vi "GUILaptop.vi"() -> ()   [LabVIEW 2016]
uses:
  Control/StreamCluster.ctl
  Control/GUICluster.ctl
panel:
  out "Joule":dbl
  out "Rundenzeit":T1
  out "stop 2":bool
  in  "Start":bool
  in  "Stop":bool
  in  "Geschwindigkeit multiplikator":dbl(knob)=0.039196582802747515 scale=0.0..1.0
  out "Linefollow-Array":bool[](array[boolean])
  out "Geschwindigkeit [m/s]":dbl(knob) scale=0.0..4.5
  out "schräg L":dbl format="%#_3g"
  out "schräge R":dbl format="%#_3g"
  out "Strom [A]":dbl(graph)
  out "rechts":dbl format="%#_3g"
  out "links":dbl format="%#_3g"
  out "gerade L":dbl format="%#_3g"
  out "gerade R":dbl format="%#_3g"
  # "Minimum"
  # "Gesamt"
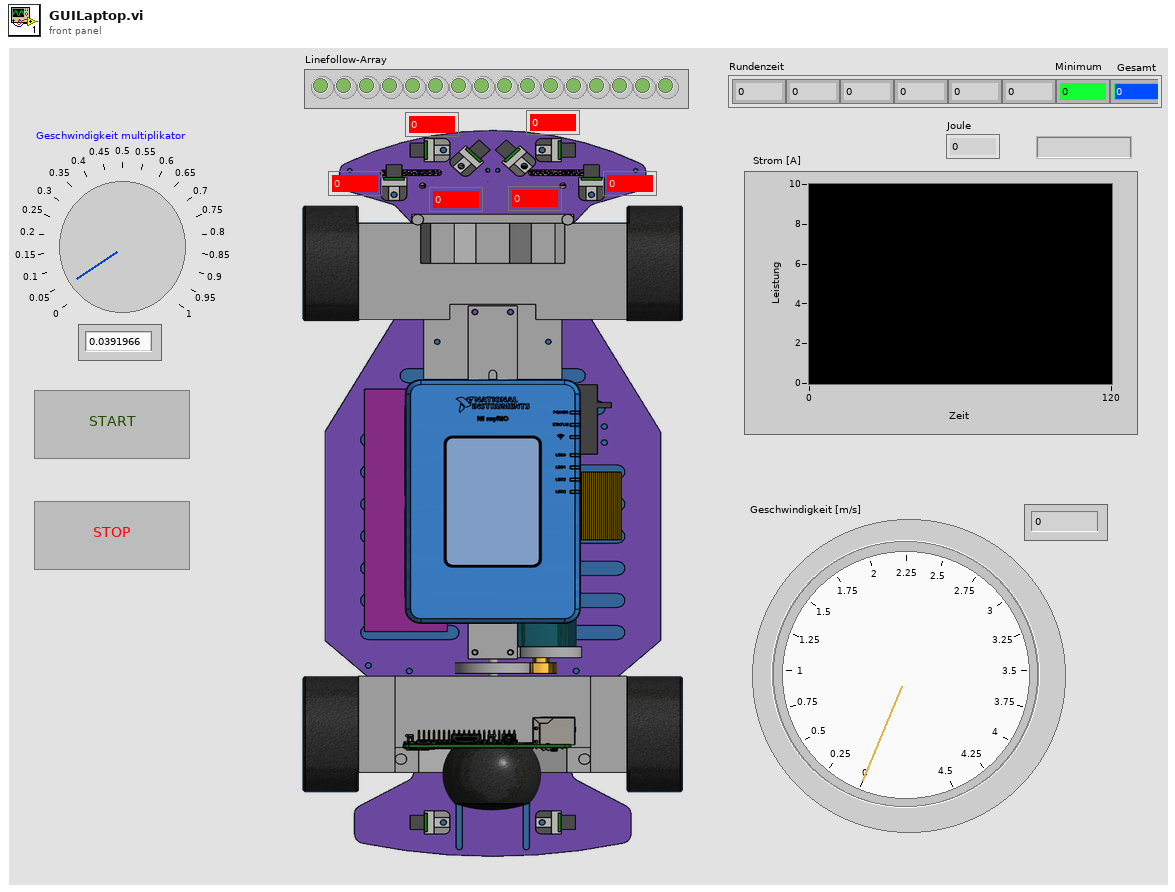
[diagram p1: front panel]
types:
  T1 = cluster{"Rundenzeit[0]":dbl, "Rundenzeit[1]":dbl, "Rundenzeit[2]":dbl, "Rundenzeit[3]":dbl, "Rundenzeit[4]":dbl, "Rundenzeit[5]":dbl, "Rundenzeit[6]":dbl, "Rundenzeit[7]":dbl, "Rundenzeit[7] 2":dbl}
  T2 = typedef "StreamCluster.ctl" = cluster{"IRSensoren":dbl[], "LineArray":bool[], "Rundenzeit":dbl[], "Drehzahl":dbl, "Leistung":dbl, "Joule":dbl}
  T3 = cluster{"Rundenzeit[0]":dbl, "Rundenzeit[1]":dbl, "Rundenzeit[2]":dbl, "Rundenzeit[3]":dbl, "Rundenzeit[4]":dbl, "Rundenzeit[5]":dbl, "Rundenzeit[6]":dbl, "Rundenzeit[7]":dbl, "Rundenzeit[8]":dbl}
  T4 = typedef "GUICluster.ctl" = cluster{"Geschwindigkeitsmultiplikator":dbl, "Stop":bool, "Start":bool}
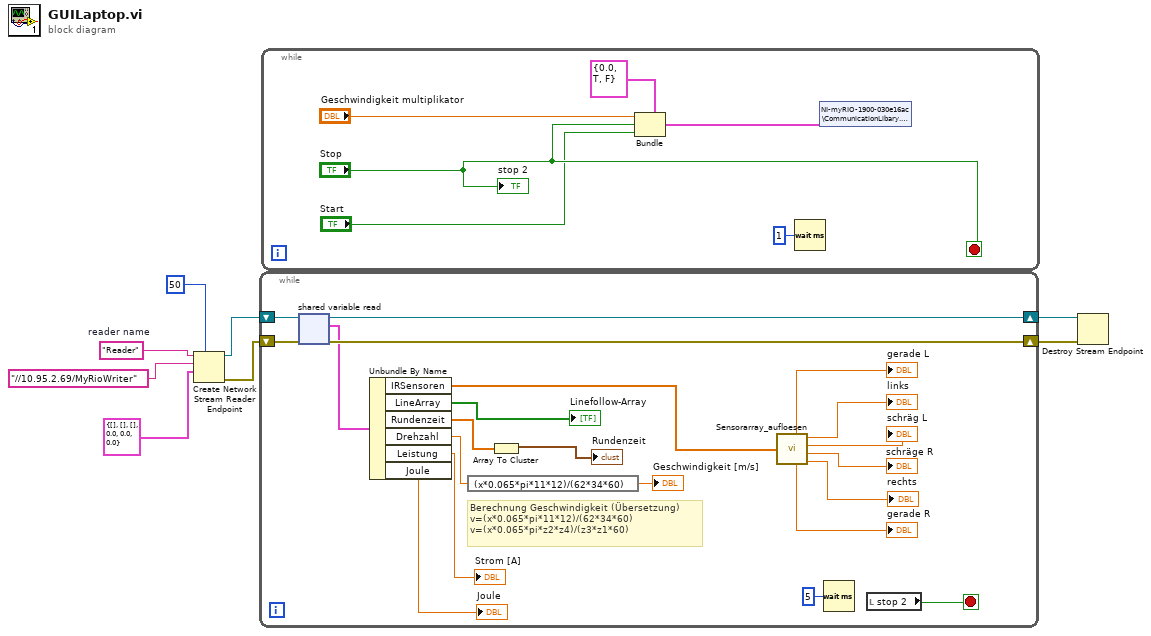
[diagram p0: block diagram]
diagram:
  w4 = "Reader"  # reader name
  n1 = Create Network Stream Reader Endpoint(7:50 ("reader buffer size"), 9:T2 {"IRSensoren"=[], "LineArray"=[], "Rundenzeit"=[], "Drehzahl"=0.0, "Leistung"=0.0, "Joule"=0.0} ("Cluster"), 10:"//10.95.2.69/MyRioWriter" ("writer url"), 11:w4) -> (0:w7:errorcluster, 3:w8:refnum<k21>)  [unwired: 3 in]
  n2 = while {
    shift-right: [w19] -> w6
    shift-left: w8 -> [w21]
    shift-right: [w18] -> w5
    shift-left: w7 -> [w20]
    stop <- w22 stop-if-true
    # "Berechnung Geschwindigkeit (Übersetzung)\nv=(x*0.065*pi*11*12)/(62*34*60)\nv=(x*0.065*pi*z2*z4)/(z3*z1*60)"
    n3 = shared-variable-read(w21, w20) -> (w19:refnum<k21>, w18:errorcluster, w17:T2)  [unwired: 1 in, 1 out]
    n4 = Unbundle By Name(w17) -> ("IRSensoren"=w14:dbl[], "LineArray"=→"Linefollow-Array":bool[], "Rundenzeit"=w11:dbl[], "Drehzahl"=w13:dbl, "Leistung"=→"Strom [A]":dbl, "Joule"=→"Joule":dbl)
    n5 = expression code="(x*0.065*pi*11*12)/(62*34*60)"(w13) -> (→"Geschwindigkeit [m/s]":dbl)
    n6 = Array To Cluster(array=w11) -> (cluster=→"Rundenzeit":T3)
    n7 = call "Sensorarray_aufloesen.vi"("Array"=w14) -> ("rechts seite"=→"rechts":dbl, "rechts geradeaus"=→"gerade R":dbl, "rechts Schräg"=→"schräge R":dbl, "Links schräg"=→"schräg L":dbl, "Links Geradeaus"=→"gerade L":dbl, "Links seite"=→"links":dbl)  [unwired: 2 in]
    n8 = Wait (ms)(milliseconds to wait=u32 5) -> ()  [unwired: 1 out]
    n9 = local read "stop 2"() -> (w22:bool)
  }
  n10 = while {
    stop <- "Stop" stop-if-true
    n11 = Bundle(cluster=T4 {"Geschwindigkeitsmultiplikator"=0.0, "Stop"=TRUE, "Start"=FALSE} ("Cluster"), "Geschwindigkeitsmultiplikator"="Geschwindigkeit multiplikator", "Stop"="Stop", "Start"="Start") -> (w30:T4)
    n12 = Wait (ms)(milliseconds to wait=u32 1) -> ()  [unwired: 1 out]
    n13 = shared-variable "NI-myRIO-1900-030e16ac\\CommunicationLibary.lvlib\\GUIInput"(w30) -> ()  [unwired: 1 in, 1 out]
    "stop 2" <- "Stop"
  }
  n14 = Destroy Stream Endpoint(8:w5, 11:w6) -> ()  [unwired: 1 out]
